vi "CheckIntercept.vi"(0 "object in":refnum<class "PositionTactic.lvclass">, 2 "GameRef":refnum<data-value>, 5 "error in (no error)":errorcluster) -> (14 "object out":refnum<class "PositionTactic.lvclass">, 16 "Intercept":bool=TRUE, 19 "error out":errorcluster)   [LabVIEW 2023, in "PositionTactic.lvclass"]
uses:
  PositionTactic.lvclass
  Game_class/Game.lvclass
  Game_class/Game.lvclass/Game.ctl
  Ball_class/Ball.lvclass/Ball.ctl
  Game_class/Read BallRef.vi
  Ball_class/Read velocityNorm.vi
  <vilib>/Analysis/_algsub.llb/Vector Norm.vi
  <vilib>/Analysis/_algsub.llb/Real Vector Norm.vi
  Ball_class/Ball.lvclass
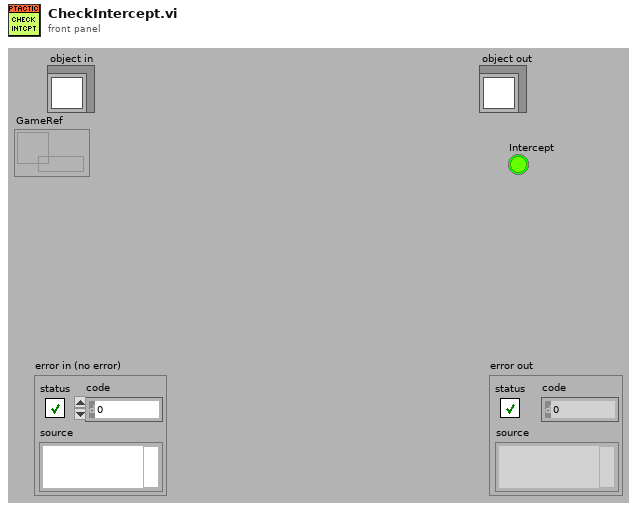
[diagram p1: front panel]
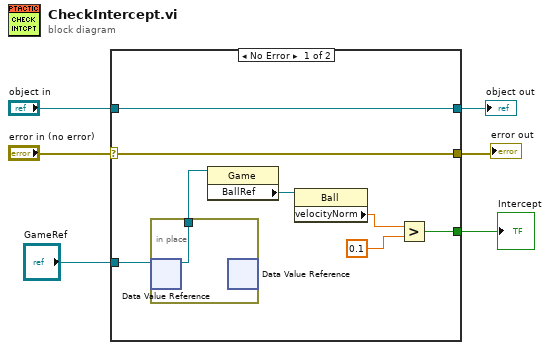
[diagram p0: block diagram]
diagram:
  n1 = case shown="No Error" "error in (no error)" {
    selector: "error in (no error)" -> [w14 w17]
    tunnel: [w14 w17] -> w5
    tunnel: [w13 w16] -> w3
    tunnel: "object in" -> [w13 w16]
    tunnel: "GameRef" -> [w12 _]
    tunnel: [w7 _] -> w1
    frame No Error {
      n2 = in-place {
        in-place-border: [w15] -> w11
        n3 = in-place-dvr #1(w12) -> (w15:refnum<class "Game.lvclass">)  [unwired: 1 out]
        n4 = in-place-dvr #1() -> ()  [unwired: 1 in, 2 out]
      }
      n5 = property class="Game"(reference=w11) -> ("BallRef"=w10:refnum<class "Ball.lvclass">)  [unwired: 1 in, 2 out]
      n6 = property class="Ball"(reference=w10) -> ("velocityNorm"=w9:dbl)  [unwired: 1 in, 2 out]
      n7 = Greater?(x=w9, y=0.1) -> (0:w7:bool)
    }
    frame Error {
    }
  }
  "error out" <- w5
  "object out" <- w3
  "Intercept" <- w1
